vi "TCP Camera Acquisition Loop.vi"(7 "Camera Controls":T1 {"VideoMode" items=["640 x 480 YUY 2 30.00 fps", "640 x 480 YUY 2 20.00 fps", "640 x 480 YUY 2 15.00 fps", "640 x 480 YUY 2 10.00 fps", "640 x 480 YUY 2 7.50 fps", "1280 x 720 YUY 2 10.00 fps", "1280 x 720 YUY 2 7.50 fps", "960 x 544 YUY 2 15.00 fps", "960 x 544 YUY 2 10.00 fps", "960 x 544 YUY 2 7.50 fps", "800 x 448 YUY 2 20.00 fps", "800 x 448 YUY 2 15.00 fps", "800 x 448 YUY 2 10.00 fps", "800 x 448 YUY 2 7.50 fps", "640 x 360 YUY 2 30.00 fps", "640 x 360 YUY 2 20.00 fps", "640 x 360 YUY 2 15.00 fps", "640 x 360 YUY 2 10.00 fps", "640 x 360 YUY 2 7.50 fps", "424 x 240 YUY 2 30.00 fps", "424 x 240 YUY 2 20.00 fps", "424 x 240 YUY 2 15.00 fps", "424 x 240 YUY 2 10.00 fps", "424 x 240 YUY 2 7.50 fps", "352 x 288 YUY 2 30.00 fps", "352 x 288 YUY 2 20.00 fps", "352 x 288 YUY 2 15.00 fps", "352 x 288 YUY 2 10.00 fps", "352 x 288 YUY 2 7.50 fps", "320 x 240 YUY 2 30.00 fps", "320 x 240 YUY 2 20.00 fps", "320 x 240 YUY 2 15.00 fps", "320 x 240 YUY 2 10.00 fps", "320 x 240 YUY 2 7.50 fps", "800 x 600 YUY 2 15.00 fps", "800 x 600 YUY 2 10.00 fps", "800 x 600 YUY 2 7.50 fps", "176 x 144 YUY 2 30.00 fps", "176 x 144 YUY 2 20.00 fps", "176 x 144 YUY 2 15.00 fps", "176 x 144 YUY 2 10.00 fps", "176 x 144 YUY 2 7.50 fps", "160 x 120 YUY 2 30.00 fps", "160 x 120 YUY 2 20.00 fps", "160 x 120 YUY 2 15.00 fps", "160 x 120 YUY 2 10.00 fps", "160 x 120 YUY 2 7.50 fps", "1280 x 800 YUY 2 10.00 fps", "640 x 480 JPEG 30.00 fps", "640 x 480 JPEG 20.00 fps", "640 x 480 JPEG 15.00 fps", "640 x 480 JPEG 10.00 fps", "640 x 480 JPEG 7.50 fps", "1280 x 720 JPEG 30.00 fps", "1280 x 720 JPEG 20.00 fps", "1280 x 720 JPEG 15.00 fps", "1280 x 720 JPEG 10.00 fps", "1280 x 720 JPEG 7.50 fps", "960 x 544 JPEG 30.00 fps", "960 x 544 JPEG 20.00 fps", "960 x 544 JPEG 15.00 fps", "960 x 544 JPEG 10.00 fps", "960 x 544 JPEG 7.50 fps", "800 x 448 JPEG 30.00 fps", "800 x 448 JPEG 20.00 fps", "800 x 448 JPEG 15.00 fps", "800 x 448 JPEG 10.00 fps", "800 x 448 JPEG 7.50 fps", "640 x 360 JPEG 30.00 fps", "640 x 360 JPEG 20.00 fps", "640 x 360 JPEG 15.00 fps", "640 x 360 JPEG 10.00 fps", "640 x 360 JPEG 7.50 fps", "800 x 600 JPEG 30.00 fps", "800 x 600 JPEG 20.00 fps", "800 x 600 JPEG 15.00 fps", "800 x 600 JPEG 10.00 fps", "800 x 600 JPEG 7.50 fps", "416 x 240 JPEG 30.00 fps", "416 x 240 JPEG 20.00 fps", "416 x 240 JPEG 15.00 fps", "416 x 240 JPEG 10.00 fps", "416 x 240 JPEG 7.50 fps", "352 x 288 JPEG 30.00 fps", "352 x 288 JPEG 20.00 fps", "352 x 288 JPEG 15.00 fps", "352 x 288 JPEG 10.00 fps", "352 x 288 JPEG 7.50 fps", "176 x 144 JPEG 30.00 fps", "176 x 144 JPEG 20.00 fps", "176 x 144 JPEG 15.00 fps", "176 x 144 JPEG 10.00 fps", "176 x 144 JPEG 7.50 fps", "320 x 240 JPEG 30.00 fps", "320 x 240 JPEG 20.00 fps", "320 x 240 JPEG 15.00 fps", "320 x 240 JPEG 10.00 fps", "320 x 240 JPEG 7.50 fps", "160 x 120 JPEG 30.00 fps", "160 x 120 JPEG 20.00 fps", "160 x 120 JPEG 15.00 fps", "160 x 120 JPEG 10.00 fps", "160 x 120 JPEG 7.50 fps"]}, 10 "Camera Number":i32, 11 "Transmission Cluster":T3) -> ()   [LabVIEW 2016]
uses:
  TCP Port Control.ctl
  Camera Settings.ctl
  38 Video Mode.ctl
  <vilib>/vision/driver/IMAQdx.llb/IMAQdx Buffer Number Mode.ctl
  <vilib>/vision/driver/NI_Vision_Acquisition_Software.lvlib
  <resource>/objmgr/imaqdx.rc
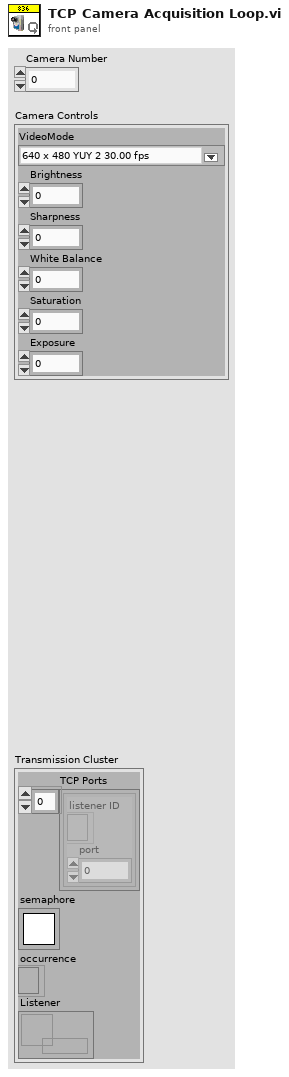
[diagram p1: front panel]
types:
  T1 = typedef "Camera Settings.ctl" = cluster{"VideoMode":T2, "Brightness":i64, "Sharpness":i64, "White Balance":i64, "Saturation":i64, "Exposure":i64}
  T2 = typedef "38 Video Mode.ctl" = u32
  T3 = typedef "TCP Port Control.ctl" = cluster{"TCP Ports":cluster{"listener ID":refnum<k5>, "port":u16}[], "semaphore":T4, "occurrence":refnum<k4>, "Listener":refnum<data-value>}
  T4 = typedef "Semaphore RefNum" = refnum<k1>
  T5 = typedef "NI_Vision_Acquisition_Software.lvlib/IMAQdx Buffer Number Mode.ctl" = enum32{"Next", "Last", "Buffer Number", "Every", "Last New"}
  T6 = cluster{"Type":u32, "Version":u32, "Flags":u32, "SerialNumberHigh":u32, "SerialNumberLow":u32, "BusType":u32, "InterfaceName":string, "VendorName":string, "ModelName":string, "CameraFileName":string, "CameraAttributeURL":string}[]
  T7 = cluster{"Type":u32, "Version":u32, "Flags":u32, "SerialNumberHigh":u32, "SerialNumberLow":u32, "BusType":u32, "InterfaceName":string, "VendorName":string, "ModelName":string, "CameraFileName":string, "CameraAttributeURL":string}
  T8 = typedef "IMAQdx.ctl" = refnum<k21>
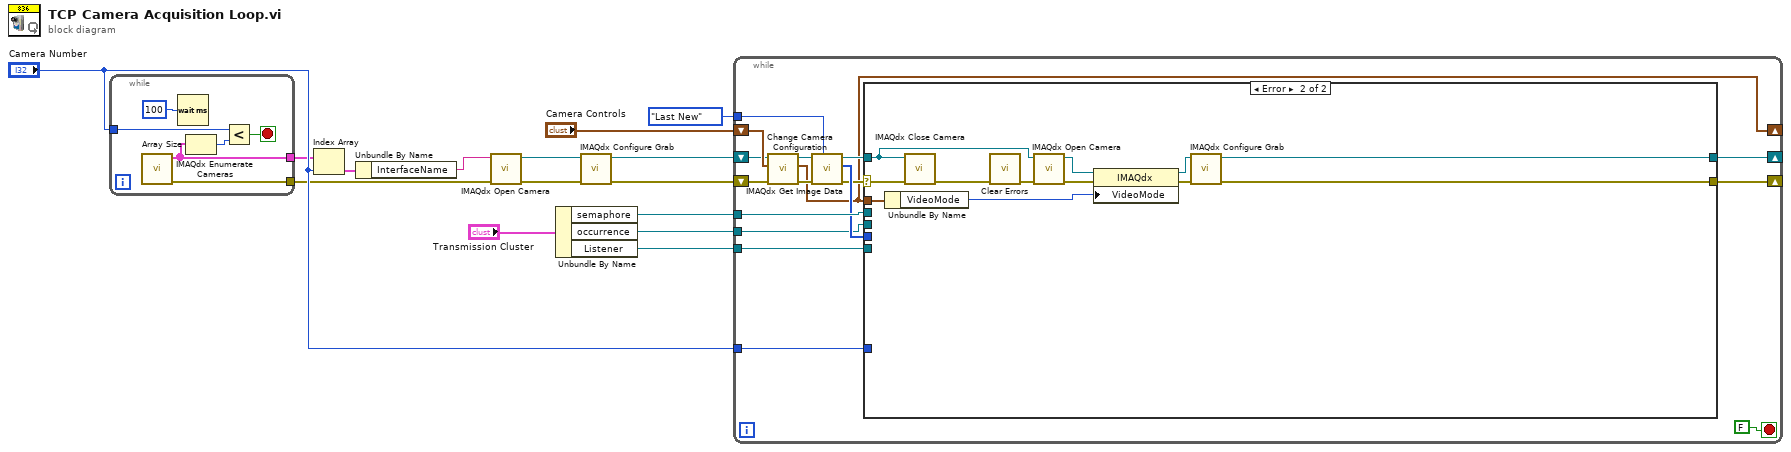
[diagram p0: block diagram]
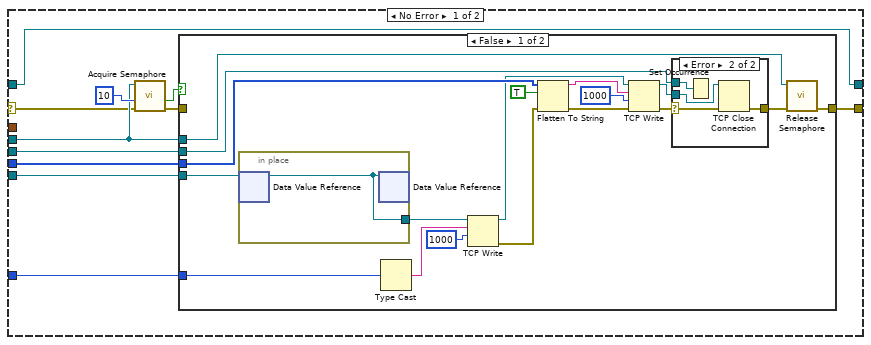
[diagram p2: hidden frame]
diagram:
  n1 = while {
    tunnel: [w20] -> w12
    tunnel: [w21] -> w7
    tunnel: "Camera Number" -> [w18]
    stop <- w17 stop-if-true
    n2 = call <vilib>:"IMAQdx Enumerate Cameras.vi"() -> ("error out"=w21:errorcluster, "Camera Information Array"=w20:T6)  [unwired: 10 in]
    n3 = Wait (ms)(milliseconds to wait=u32 100) -> ()  [unwired: 1 out]
    n4 = Array Size(array=w20) -> (size(s)=w19:i32)
    n5 = Less?(x=w18, y=w19) -> (x < y?=w17:bool)
  }
  n6 = Index Array(array=w12, index="Camera Number") -> (element=w11:T7)
  n7 = Unbundle By Name(w11) -> ("InterfaceName"=w9:string)
  n8 = call <vilib>:"IMAQdx Open Camera.vi"("error in"=w7, "Session In"=w9) -> ("error out"=w6:errorcluster, "Session Out"=w8:T8)  [unwired: 8 in]
  n9 = Unbundle By Name("Transmission Cluster") -> ("semaphore"=w3:T4, "occurrence"=w2:refnum<k4>, "Listener"=w4:refnum<data-value>)
  n10 = call <vilib>:"IMAQdx Configure Grab.vi"("error in"=w6, "Session In"=w8) -> ("error out"=w5:errorcluster, "Session Out"=w1:T8)  [unwired: 8 in]
  n11 = while {
    tunnel: w3 -> [w36]
    tunnel: IMAQdx_Buffer_Number_Mode."Last New" ("Buffer Number Mode (Next)") -> [w37]
    tunnel: w4 -> [w35]
    tunnel: "Camera Number" -> [w33]
    tunnel: w2 -> [w32]
    shift-right: [w22] -> _
    shift-left: "Camera Controls" -> [w31]
    shift-right: [w23] -> _
    shift-left: w1 -> [w30]
    shift-right: [w25] -> _
    shift-left: w5 -> [w27]
    stop <- FALSE stop-if-true
    n12 = call "Change Camera Configuration.vi"("error in (no error)"=w27, "Camera Controls"=w31, "Camera Session"=w30) -> ("error out"=w26:errorcluster, "Camera Controls Out"=w22:T1, "Session out"=w24:T8)  [unwired: 6 in]
    n13 = call <vilib>:"IMAQdx Get Image Data.vi"("Buffer Number Mode (Next)"=w37, "error in"=w26, "Session In"=w24) -> ("error out"=w29:errorcluster, "Image Data Array"=w34:u8[], "Session Out"=w28:T8)  [unwired: 5 in, 1 out]
    n14 = case shown="Error" w29 {
      selector: w29 -> [w42 w81]
      tunnel: w36 -> [w47 _]
      tunnel: w35 -> [w46 _]
      tunnel: w34 -> [w45 _]
      tunnel: w33 -> [w44 _]
      tunnel: w32 -> [w43 _]
      tunnel: w28 -> [w40 w80]
      tunnel: [w41 w79] -> w25
      tunnel: [w40 w78] -> w23
      tunnel: w22 -> [_ w75]
      frame No Error {
        n15 = call <vilib>:"Acquire Semaphore.vi"("error in (no error)"=w42, "ms timeout (-1)"=10, "semaphore"=w47) -> ("error out"=w39:errorcluster, "timed out"=w49:bool)  [unwired: 2 in, 1 out]
        n16 = case shown="False" w49 {
          tunnel: w47 -> [w63 _]
          tunnel: w46 -> [w62 _]
          tunnel: w45 -> [w60 _]
          tunnel: w44 -> [w59 _]
          tunnel: w43 -> [w54 _]
          tunnel: [w52 _] -> w41
          tunnel: w39 -> [_ _]
          frame False {
            n17 = in-place {
              in-place-border: [w73] -> w61
              n18 = in-place-dvr #1(w62) -> (w73:refnum<k5>)  [unwired: 1 out]
              n19 = in-place-dvr #1(w73) -> ()  [unwired: 2 out]
            }
            n20 = Type Cast(x=w59) -> (*(type *) &x=w58:string)  [unwired: 1 in]
            n21 = TCP Write(connection ID=w61, data in=w58, 9:1000 ("timeout ms (25000)")) -> (connection ID out=w51:refnum<k5>, error out=w64:errorcluster)  [unwired: 1 in, 1 out]
            n22 = Flatten To String(anything=w60, prepend array or string size? (T)=TRUE, error in (no error)=w64) -> (data string=w66:string, error out=w67:errorcluster)  [unwired: 1 in, 1 out]
            n23 = TCP Write(connection ID=w51, data in=w66, error in (no error)=w67, 9:1000 ("timeout ms (25000)")) -> (connection ID out=w50:refnum<k5>, error out=w55:errorcluster)  [unwired: 1 out]
            n24 = case shown="Error" w55 {
              selector: w55 -> [w68 w70]
              tunnel: w54 -> [_ w72]
              tunnel: [w68 w69] -> w53
              tunnel: w50 -> [_ w71]
              frame No Error {
              }
              frame Error {
                n25 = Set Occurrence(w72) -> ()
                n26 = TCP Close Connection(connection ID=w71, error in (no error)=w70) -> (error out=w69:errorcluster)  [unwired: 1 in, 1 out]
              }
            }
            n27 = call <vilib>:"Release Semaphore.vi"("error in (no error)"=w53, "semaphore"=w63) -> ("error out"=w52:errorcluster)  [unwired: 4 in, 1 out]
          }
          frame True {
          }
        }
      }
      frame Error {
        n28 = Unbundle By Name(w75) -> ("VideoMode"=w74:T2)
        n29 = call <vilib>:"IMAQdx Close Camera.vi"("error in"=w81, "Session In"=w80) -> ("error out"=w85:errorcluster)  [unwired: 9 in]
        n30 = call <vilib>:"Clear Errors.vi"("error in (no error)"=w85) -> ("error out"=w84:errorcluster)  [unwired: 5 in, 1 out]
        n31 = call <vilib>:"IMAQdx Open Camera.vi"("error in"=w84, "Session In"=w80) -> ("error out"=w83:errorcluster, "Session Out"=w77:T8)  [unwired: 8 in]
        n32 = property class="IMAQdx"(reference=w77, error in=w83, "VideoMode"=w74) -> (reference out=w76:T8, error out=w82:errorcluster)
        n33 = call <vilib>:"IMAQdx Configure Grab.vi"("error in"=w82, "Session In"=w76) -> ("error out"=w79:errorcluster, "Session Out"=w78:T8)  [unwired: 8 in]
      }
    }
  }
